vi "Wait.vi"(7 "Name":string="Wait", 11 "Time (ms)":u32) -> (3 "Node Out":refnum<class "abs_Node.lvclass">)   [LabVIEW 2021, in "BT.lvlib"]
uses:
  BT.lvlib
  abs_Node/abs_Node.lvclass
  Wait/Wait.lvclass
  C:/Users/Tim/Documents/LabVIEW/2021/Behaviour Tree/abs_Node/abs_Node.lvclass
  Wait/Wait.lvclass/Wait.ctl
  abs_Node/abs_Node.lvclass/abs_Node.ctl
  Wait/Properties/Write Time (ms).vi
  abs_Node/Properties/Write Name.vi
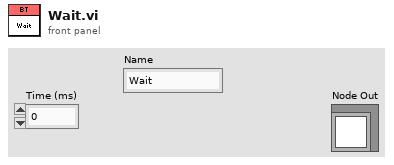
[diagram p1: front panel]
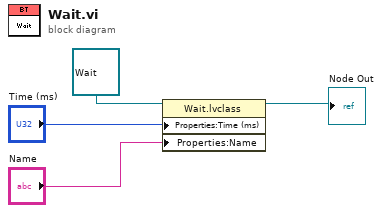
[diagram p0: block diagram]
diagram:
  n1 = property class="Wait.lvclass"(reference=refnum<class "Wait.lvclass"> refnum ("BT.lvlib:Wait.lvclass"), "Properties:Time (ms)"="Time (ms)", "Properties:Name"="Name") -> (reference out=→"Node Out":refnum<class "Wait.lvclass">)  [unwired: 1 in, 1 out]
